vi "KM101_IdentifyHarware.vi"(10 "reference in":refnum<k7>) -> (2 "reference out":refnum<k7>)   [LabVIEW 2018, in "KIM101lib.lvlib"]
uses:
  KIM101lib.lvlib
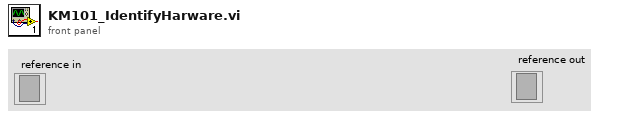
[diagram p1: front panel]
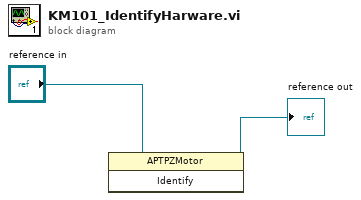
[diagram p0: block diagram]
diagram:
  n1 = invoke class="APTPZMotor" method="Identify"(reference="reference in") -> (reference out=→"reference out":refnum<k7>)  [unwired: 2 in, 2 out]
